vi "setName.vi"(8 "error in (no error)":errorcluster, 10 "Name":string, 11 "tBSONElement in":refnum<class "tBSONElement.lvclass">) -> (0 "error out":errorcluster, 3 "tBSONElement out":refnum<class "tBSONElement.lvclass">)   [LabVIEW 2013, in "BSON.lvlib" / "tBSONElement.lvclass"]
uses:
  tBSONElement.lvclass
  tBSONElement.lvclass/tBSONElement.ctl
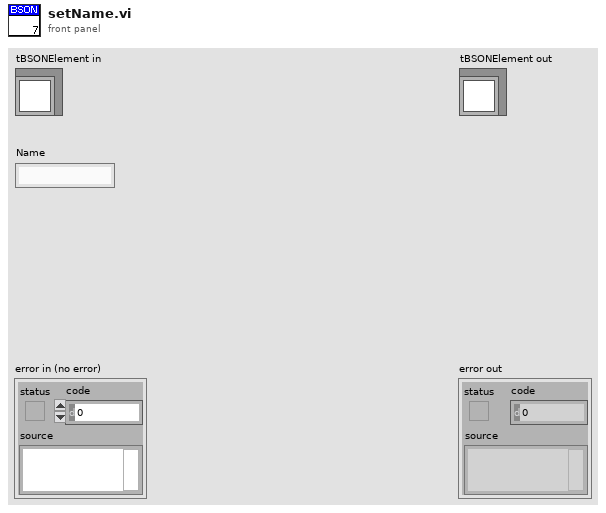
[diagram p1: front panel]
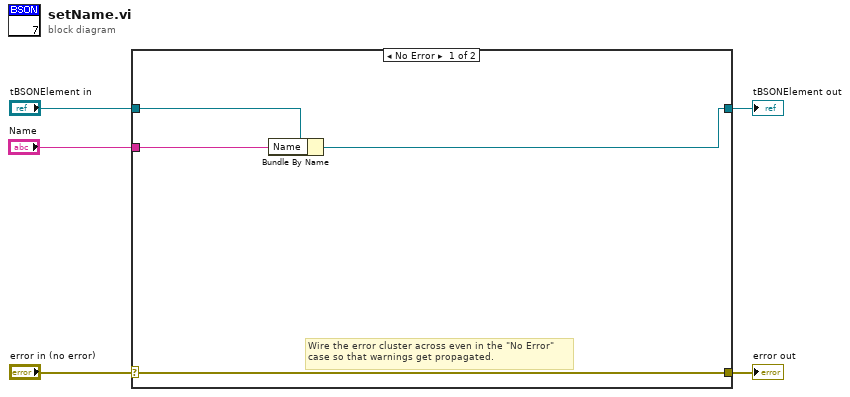
[diagram p0: block diagram]
diagram:
  n1 = case shown="No Error" "error in (no error)" {
    selector: "error in (no error)" -> [w9 w11]
    tunnel: [w9 w11] -> w4
    tunnel: [w7 w10] -> w2
    tunnel: "tBSONElement in" -> [w8 w10]
    tunnel: "Name" -> [w6 _]
    frame No Error {
      # "Wire the error cluster across even in the \"No Error\"\ncase so that warnings get propagated."
      n2 = Bundle By Name(cluster=w8, "Name"=w6) -> (w7:refnum<class "tBSONElement.lvclass">)
    }
    frame Error {
    }
  }
  "error out" <- w4
  "tBSONElement out" <- w2
